vi "Create Type Definition.vi"(8 "error in (no error)":errorcluster) -> (0 "error out":errorcluster, 3 "TypeDef VI out":refnum<vi>)   [LabVIEW 2019, in "gRPC Scripting Tools.lvlib"]
uses:
  gRPC Scripting Tools.lvlib
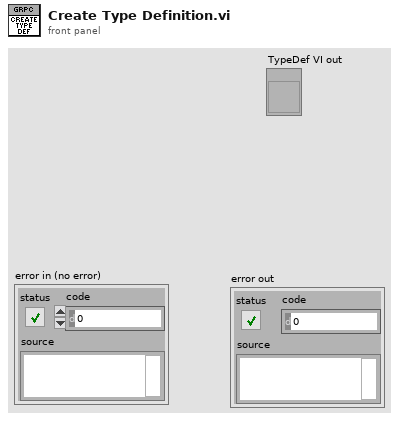
[diagram p1: front panel]
types:
  T1 = enum32{"not a control VI", "control", "typedef", "strict typedef"}
  T2 = enum32{"invalid VI type", "Standard VI", "Control VI", "Global VI", "Polymorphic VI", "Configuration VI", "SubSystem", "Facade VI", "Method VI", "Statechart Diagram VI"}
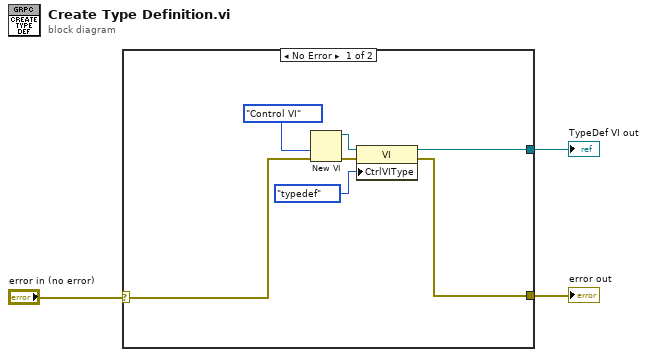
[diagram p0: block diagram]
diagram:
  n1 = case shown="No Error" "error in (no error)" {
    selector: "error in (no error)" -> [w4 w11]
    tunnel: [w10 w11] -> w3
    tunnel: [w9 _] -> w2
    frame No Error {
      n2 = New VI(8:w4, 9:T2."Control VI" ("vi type (standard vi)")) -> (0:w7:errorcluster, 3:w8:refnum<vi>)  [unwired: 5 in]
      n3 = property class="VI"(reference=w8, error in=w7, "CtrlVIType"=T1."typedef" ("Control VI Type")) -> (reference out=w9:refnum<vi>, error out=w10:errorcluster)
    }
    frame Error {
    }
  }
  "error out" <- w3
  "TypeDef VI out" <- w2
